vi "Initialize.vi"(3 "error in":errorcluster) -> (0 "error out":errorcluster, 2 "ref out":refnum<k7>)   [LabVIEW 2010]
panel:
  in  "IPCamX":refnum<k7>(container)
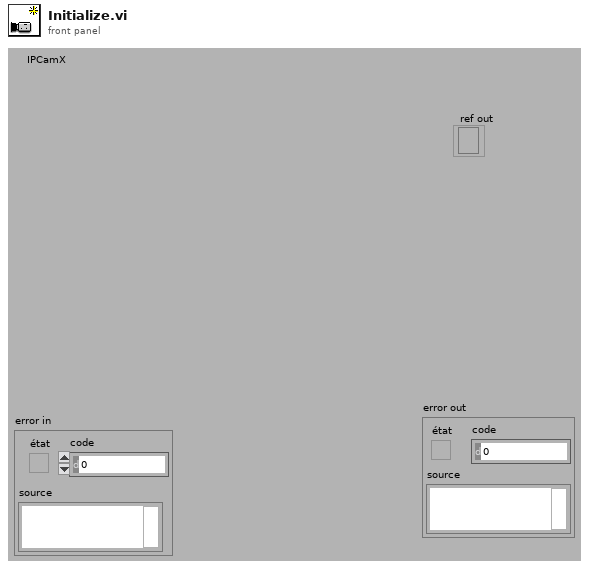
[diagram p1: front panel]
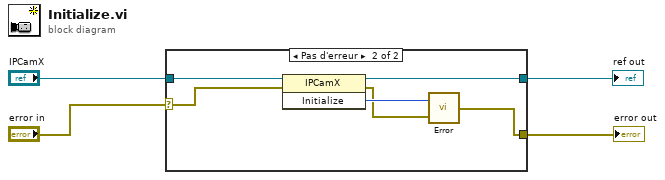
[diagram p0: block diagram]
diagram:
  n1 = case shown="Pas d'erreur" "error in" {
    selector: "error in" -> [w5 w12]
    tunnel: [w5 w7] -> w4
    tunnel: [w6 w10] -> w3
    tunnel: "IPCamX" -> [w6 w11]
    frame Error {
    }
    frame No Error {
      n2 = invoke class="IPCamX" method="Initialize"(reference=w11, error in=w12) -> (reference out=w10:refnum<k7>, error out=w8:errorcluster, "Initialize"=w9:i32)  [unwired: 1 in]
      n3 = call "Error.vi"("error in"=w8, "code"=w9) -> ("error out"=w7:errorcluster)
    }
  }
  "error out" <- w4
  "ref out" <- w3
